vi "Rohde & Schwarz VNA Read Learn String.vi"(7 "Rohde & Schwarz VNA":T1, 8 "error in (no error)":errorcluster, 11 "VISA Resource Name":refnum<visa-resource-name>) -> (0 "error out":errorcluster, 2 "Learn String":string, 3 "dup VISA Resource Name":refnum<visa-resource-name>)   [LabVIEW 2011]
uses:
  TypeDefs/Rohde & Schwarz VNA Instrument Info.ctl
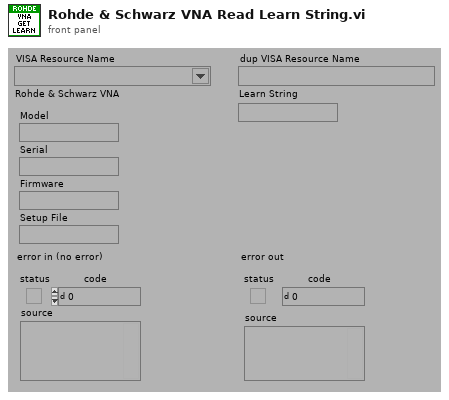
[diagram p1: front panel]
types:
  T1 = typedef "Rohde & Schwarz VNA Instrument Info.ctl" = cluster{"Model":string, "Serial":string, "Firmware":string, "Setup File":string}
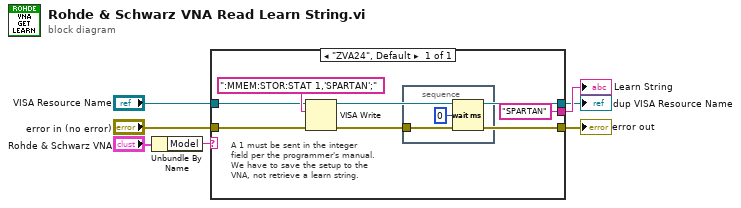
[diagram p0: block diagram]
diagram:
  n1 = Unbundle By Name("Rohde & Schwarz VNA") -> ("Model"=w1:string)
  n2 = case shown="\"ZVA24\", Default" w1 {
    tunnel: "VISA Resource Name" -> [w12]
    tunnel: ["SPARTAN"] -> w6
    tunnel: "error in (no error)" -> [w11]
    tunnel: [w8] -> w4
    tunnel: [w10] -> w3
    frame "ZVA24", Default {
      # "A 1 must be sent in the integer\nfield per the programmer's manual.\nWe have to save the setup to the\nVNA, not retrieve a learn string."
      n3 = VISA Write(VISA resource name=w12, write buffer=":MMEM:STOR:STAT 1,'SPARTAN';", error in (no error)=w11) -> (VISA resource name out=w10:refnum<visa-resource-name>, error out=w8:errorcluster)  [unwired: 1 out]
      n4 = stacked-sequence {
        tunnel: w8 -> [_]
        frame #0 {
          n5 = Wait (ms)(milliseconds to wait=u32 0) -> ()  [unwired: 1 out]
        }
      }
    }
  }
  "error out" <- w4
  "dup VISA Resource Name" <- w3
  "Learn String" <- w6
